vi "R-S触发器功能测试.vi"() -> ()   [LabVIEW 2018]
panel:
  in  "确定按钮":bool
  out "Q`":bool
  out "Q":bool
  in  "S`":bool
  in  "R`":bool
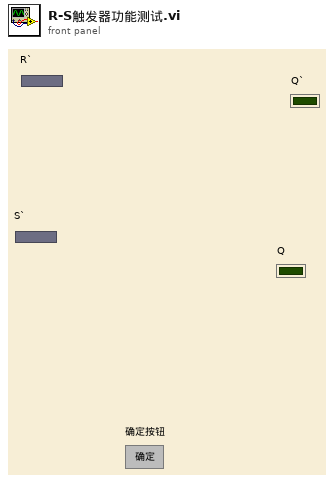
[diagram p1: front panel]
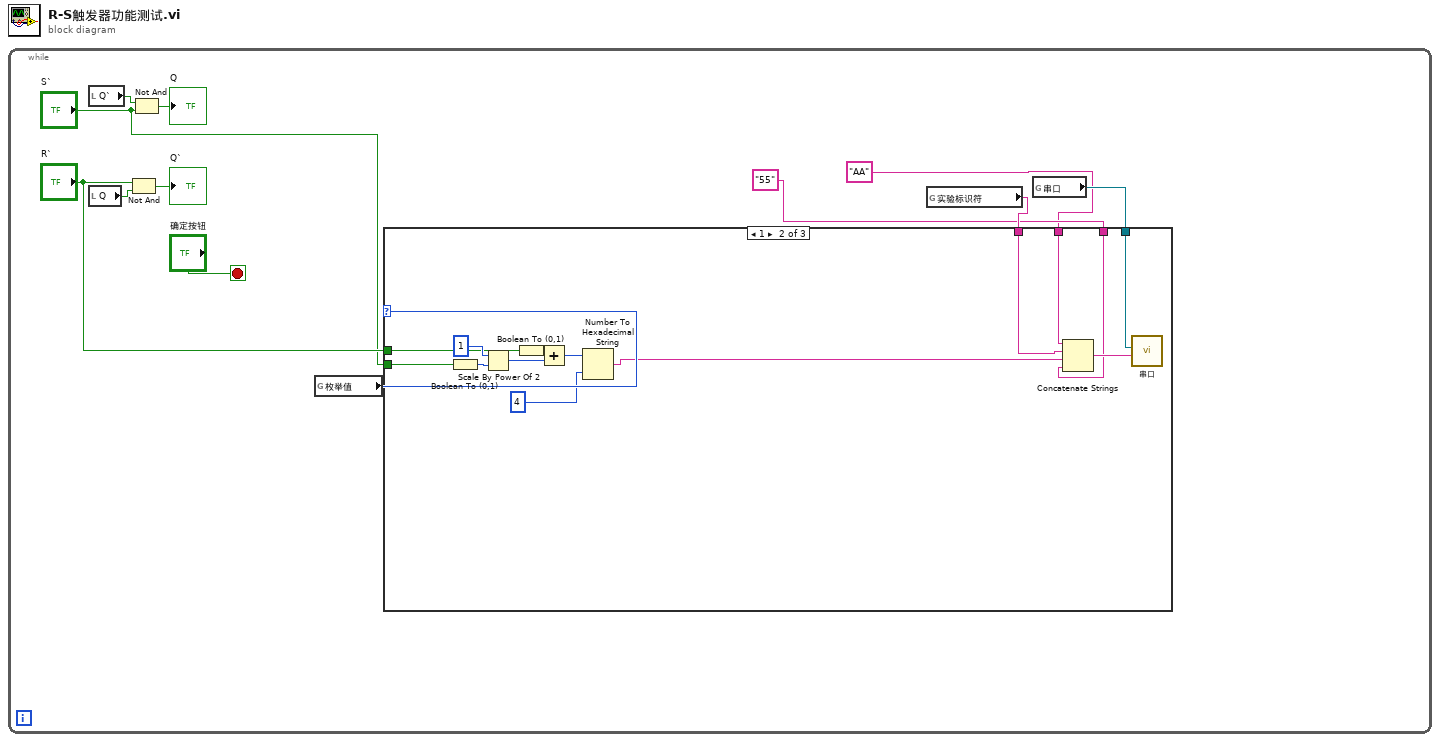
[diagram p0: block diagram]
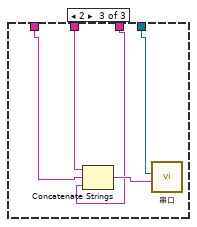
[diagram p3: hidden frame]
diagram:
  n1 = while {
    stop <- "确定按钮" stop-if-true
    n2 = local read "Q`"() -> (w11:bool)
    n3 = local read "Q"() -> (w9:bool)
    n4 = Not And(1:w9, 2:"R`") -> (0:→"Q`":bool)
    n5 = Not And(1:"S`", 2:w11) -> (0:→"Q":bool)
    n6 = global read "全局变量.vi" "枚举值"() -> (w7:i8)
    n7 = global read "全局变量.vi" "实验标识符"() -> (w5:string)
    n8 = global read "全局变量.vi" "串口"() -> (w6:refnum<visa-resource-name>)
    n9 = case shown="1" w7 {
      tunnel: "S`" -> [_ w21 _]
      tunnel: "R`" -> [_ w20 _]
      tunnel: w6 -> [_ w19 w29]
      tunnel: w5 -> [_ w18 w30]
      tunnel: "55" -> [_ w17 w27]
      tunnel: "AA" -> [_ w16 w28]
      frame 0, Default {
      }
      frame 1 {
        n10 = Boolean To (0,1)(Boolean=w21) -> (0, 1=w23:i16)
        n11 = Scale By Power Of 2(n=1, x=w23) -> (x*2^n=w24:i16)
        n12 = Boolean To (0,1)(Boolean=w20) -> (0, 1=w25:i16)
        n13 = Add(x=w25, y=w24) -> (x+y=w15:i16)
        n14 = Number To Hexadecimal String(1:4, 2:w15) -> (0:w13:string)
        n15 = Concatenate Strings(w16, w18, w13, w17) -> (w26:string)
        n16 = call "串口.vi"("字符串"=w26, "VISA resource name"=w19) -> ()  [unwired: 10 in]
      }
      frame 2 {
        n17 = Concatenate Strings(w28, w30, w27) -> (w31:string)
        n18 = call "串口.vi"("字符串"=w31, "VISA resource name"=w29) -> ()  [unwired: 10 in]
      }
    }
  }
